vi "Extract Data Optional.vi"(8 "error in (no error)":errorcluster caption="entrée d'erreur (pas d'erreur)", 11 "Parsing Data RADIO_ERP1 en entrée":refnum<class "Parsing Data RADIO_ERP1.lvclass">) -> (0 "error out":errorcluster caption="sortie d'erreur", 3 "Parsing Data RADIO_ERP1 en sortie":refnum<class "Parsing Data RADIO_ERP1.lvclass">)   [LabVIEW 2020, in "Library Instrument & Equipement.lvlib" / "Library UART.lvlib" / "Parsing Data RADIO_ERP1.lvclass"]
uses:
  Parsing Data RADIO_ERP1.lvclass
  C:/Users/ngarcin/OneDrive - Altyor/Standard TB/Class/UART/UART Enocean/Parsing Data Enocean (Default)/Parsing Data Enocean (Default).lvclass
  Parsing Data RADIO_ERP1.lvclass/Parsing Data RADIO_ERP1.ctl
  Commun VI/Library Commun.lvlib
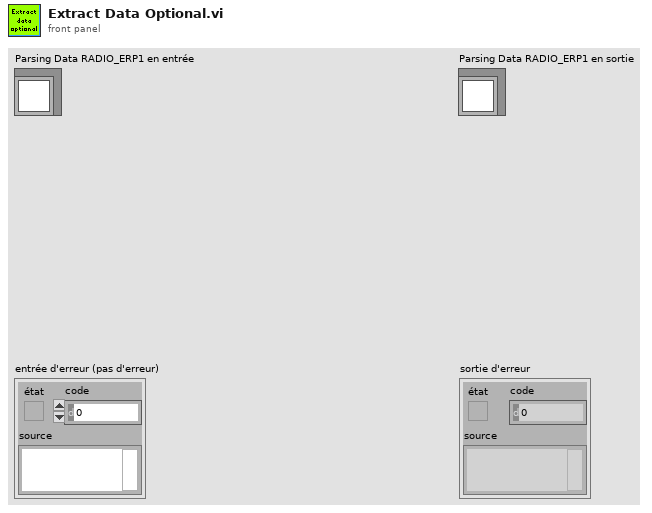
[diagram p1: front panel]
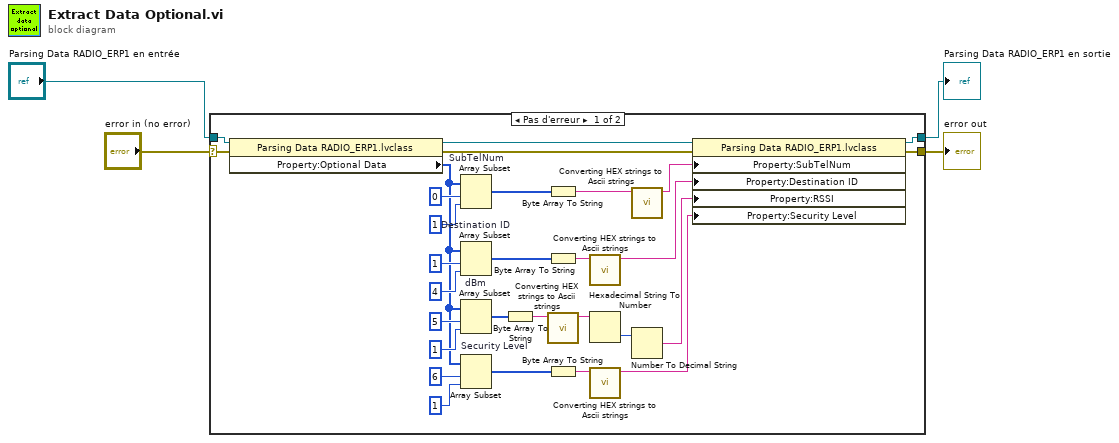
[diagram p0: block diagram]
diagram:
  n1 = case shown="Pas d'erreur" "error in (no error)" {
    selector: "error in (no error)" -> [w8 w35]
    tunnel: [w7 w35] -> w3
    tunnel: [w27 w34] -> w1
    tunnel: "Parsing Data RADIO_ERP1 en entrée" -> [w33 w34]
    frame No Error {
      n2 = property class="Parsing Data RADIO_ERP1.lvclass"(reference=w33, error in=w8) -> (reference out=w32:refnum<class "Parsing Data RADIO_ERP1.lvclass">, error out=w9:errorcluster, "Property:Optional Data"=w13:u8[])
      n3 = Array Subset "SubTelNum"(array=w13, index=0 ("indice"), length=1 ("longueur")) -> (w26:u8[])
      n4 = Array Subset "Destination ID"(array=w13, index=1 ("indice"), length=4 ("indice")) -> (w23:u8[])
      n5 = Array Subset "dBm"(array=w13, index=5 ("indice"), length=1 ("longueur")) -> (w18:u8[])
      n6 = Array Subset "Security Level"(array=w13, index=6 ("indice"), length=1 ("longueur")) -> (w12:u8[])
      n7 = Byte Array To String(unsigned byte array=w18) -> (string=w17:string)
      n8 = Byte Array To String(unsigned byte array=w26) -> (string=w25:string)
      n9 = Byte Array To String(unsigned byte array=w23) -> (string=w22:string)
      n10 = call "Converting HEX strings to Ascii strings.vi"("chaîne IN"=w17) -> ("Chaîne OUT"=w16:string)  [unwired: 9 in, 1 out]
      n11 = Byte Array To String(unsigned byte array=w12) -> (string=w15:string)
      n12 = call "Converting HEX strings to Ascii strings.vi"("chaîne IN"=w22) -> ("Chaîne OUT"=w21:string)  [unwired: 9 in, 1 out]
      n13 = Hexadecimal String To Number(string=w16) -> (number=w6:u32)  [unwired: 2 in, 1 out]
      n14 = call "Converting HEX strings to Ascii strings.vi"("chaîne IN"=w15) -> ("Chaîne OUT"=w14:string)  [unwired: 9 in, 1 out]
      n15 = call "Converting HEX strings to Ascii strings.vi"("chaîne IN"=w25) -> ("Chaîne OUT"=w24:string)  [unwired: 9 in, 1 out]
      n16 = Number To Decimal String(number=w6) -> (decimal integer string=w5:string)  [unwired: 1 in]
      n17 = property class="Parsing Data RADIO_ERP1.lvclass"(reference=w32, error in=w9, "Property:SubTelNum"=w24, "Property:Destination ID"=w21, "Property:RSSI"=w5, "Property:Security Level"=w14) -> (reference out=w27:refnum<class "Parsing Data RADIO_ERP1.lvclass">, error out=w7:errorcluster)
    }
    frame Error {
    }
  }
  "error out" <- w3
  "Parsing Data RADIO_ERP1 en sortie" <- w1
